vi "construct send command.vi"(10 "GCode":string) -> (3 "SendCommand":string)   [LabVIEW 2014, in "HPCNC.lvlib"]
uses:
  HPCNC.lvlib
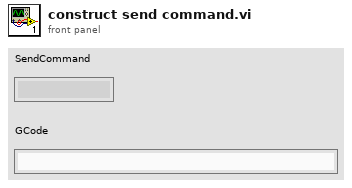
[diagram p1: front panel]
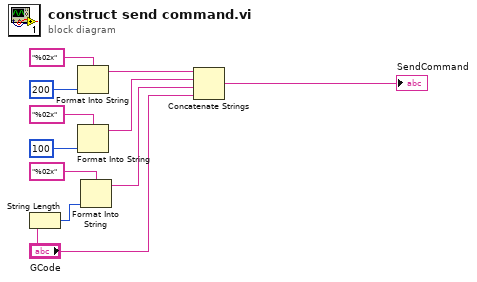
[diagram p0: block diagram]
diagram:
  n1 = String Length(string="GCode") -> (length=w5:i32)
  n2 = Format Into String(format string="%02x", 200) -> (resulting string=w9:string)  [unwired: 2 in, 1 out]
  n3 = Format Into String(format string="%02x", i8 100 ("input 1")) -> (resulting string=w7:string)  [unwired: 2 in, 1 out]
  n4 = Format Into String(format string="%02x", w5) -> (resulting string=w4:string)  [unwired: 2 in, 1 out]
  n5 = Concatenate Strings(w9, w7, w4, "GCode") -> (→"SendCommand":string)
